vi "Get Tree Children.vi"(8 "error in (no error)":errorcluster, 9 "Parent Tag":string, 10 "Child Tags In":string[](array[string]), 11 "File Contents Tree":refnum<vi>) -> (0 "error out":errorcluster, 2 "Child Tags Out":string[](array[string]))   [LabVIEW 2017, in "XTree.xctl"]
doc: "Recursively finds all of the tree locations without children under a given location."
uses:
  <vilib>/addons/_NIFileIO/XTree/XTree.xctl
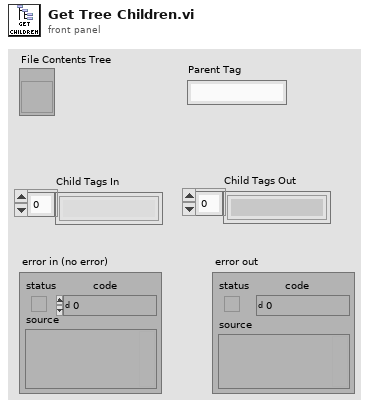
[diagram p1: front panel]
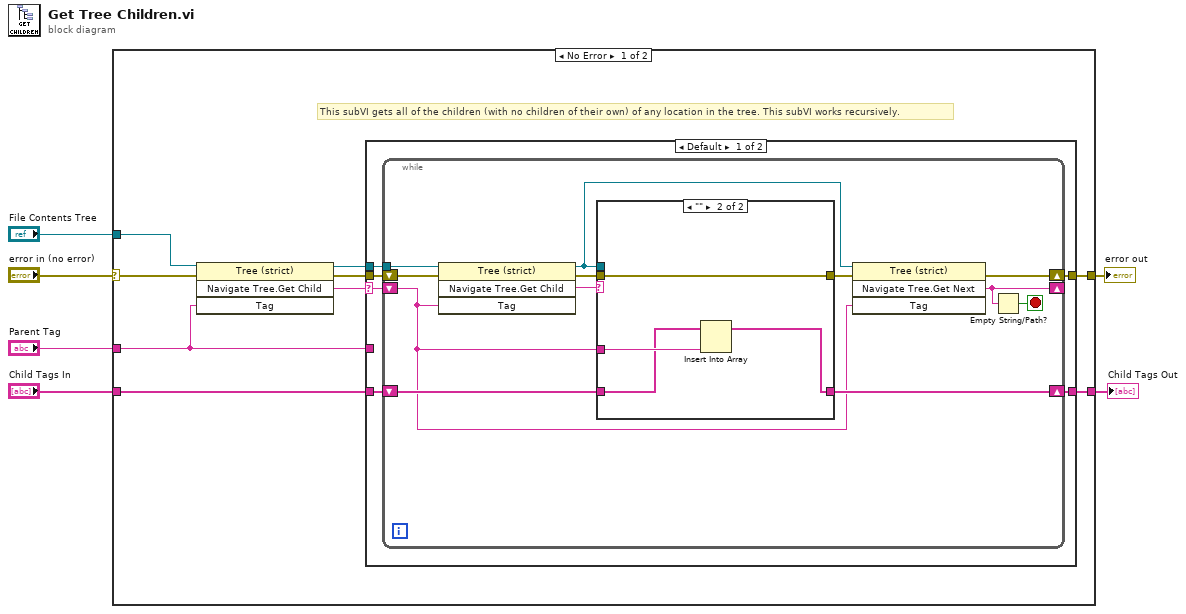
[diagram p0: block diagram]
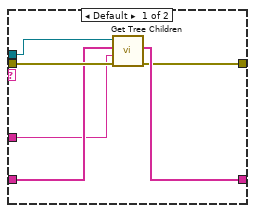
[diagram p2: hidden frame]
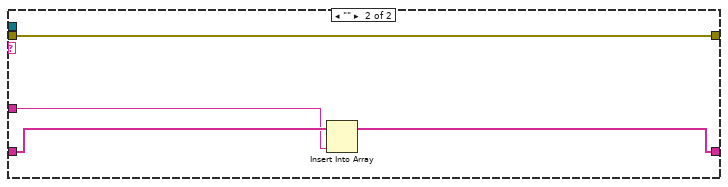
[diagram p3: hidden frame]
diagram:
  n1 = case shown="No Error" "error in (no error)" {
    selector: "error in (no error)" -> [w11 w49]
    tunnel: [w13 w49] -> w6
    tunnel: "Child Tags In" -> [w10 w48]
    tunnel: [w9 w48] -> w3
    tunnel: "Parent Tag" -> [w8 _]
    tunnel: "File Contents Tree" -> [w7 _]
    frame No Error {
      # "This subVI gets all of the children (with no children of their own) of any location in the tree. This subVI works recursively."
      n2 = invoke class="Tree (strict)" method="Navigate Tree.Get Child"(reference=w7, error in=w11, "Tag"=w8) -> (reference out=w12:refnum<vi>, error out=w14:errorcluster, "Navigate Tree:Get Child"=w15:string)  [unwired: 1 in, 1 out]
      n3 = case shown="Default" w15 {
        selector: w15 -> [w20 _]
        tunnel: w14 -> [w19 w47]
        tunnel: [w18 w47] -> w13
        tunnel: w10 -> [w17 w46]
        tunnel: [w16 w44] -> w9
        tunnel: w12 -> [w21 _]
        tunnel: w8 -> [_ w45]
        frame Default {
          n4 = while {
            tunnel: w21 -> [w30]
            shift-right: [w32] -> _
            shift-left: w20 -> [w25]
            shift-right: [w31] -> w18
            shift-left: w19 -> [w29]
            shift-right: [w26] -> w16
            shift-left: w17 -> [w27]
            stop <- w33 stop-if-true
            n5 = invoke class="Tree (strict)" method="Navigate Tree.Get Child"(reference=w30, error in=w29, "Tag"=w25) -> (reference out=w23:refnum<vi>, error out=w24:errorcluster, "Navigate Tree:Get Child"=w28:string)  [unwired: 1 in, 1 out]
            n6 = case shown="\"\"" w28 {
              tunnel: w27 -> [w37 w42]
              tunnel: [w35 w41] -> w26
              tunnel: w25 -> [w36 w43]
              tunnel: w24 -> [w39 w40]
              tunnel: w23 -> [w38 _]
              tunnel: [w34 w40] -> w22
              frame Default {
                n7 = call <vilib>:"Get Tree Children.vi"("error in (no error)"=w39, "Parent Tag"=w36, "Child Tags In"=w37, "File Contents Tree"=w38) -> ("error out"=w34:errorcluster, "Child Tags Out"=w35:string[])  [unwired: 6 in]
              }
              frame "" {
                n8 = Insert Into Array(array=w42, new element=w43) -> (w41:string[])  [unwired: 1 in]
              }
            }
            n9 = invoke class="Tree (strict)" method="Navigate Tree.Get Next"(reference=w23, error in=w22, "Tag"=w25) -> (error out=w31:errorcluster, "Navigate Tree:Get Next Item"=w32:string)  [unwired: 1 in, 2 out]
            n10 = Empty String/Path?(string/path=w32) -> (empty?=w33:bool)
          }
        }
        frame "" {
          n11 = Insert Into Array(array=w46, new element=w45) -> (w44:string[])  [unwired: 1 in]
        }
      }
    }
    frame Error {
    }
  }
  "error out" <- w6
  "Child Tags Out" <- w3
